vi "Configure Serial.vi"(8 "error in (no error)":errorcluster, 10 "Baud (115200)":u32=115200, 11 "VISA resource name in":refnum<visa-resource-name>) -> (0 "error out":errorcluster, 3 "VISA resource name":refnum<visa-resource-name>)   [LabVIEW 2023, in "CTI-Visa.lvlib"]
uses:
  CTI-Visa.lvlib
  <vilib>/Instr/_visa.llb/VISA Configure Serial Port (Instr).vi
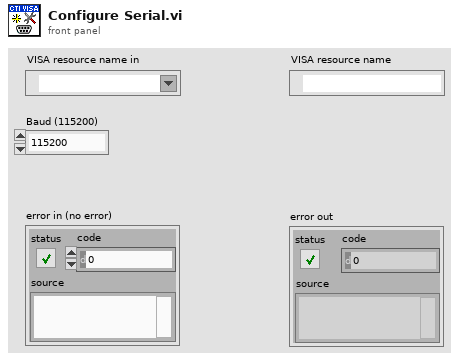
[diagram p1: front panel]
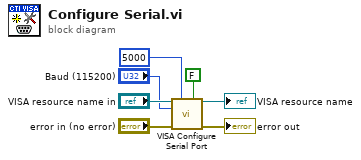
[diagram p0: block diagram]
diagram:
  n1 = call-poly "VISA Configure Serial Port"("VISA resource name"="VISA resource name in", "timeout (10sec)"=u32 5000, "Enable Termination\nChar (T)"=FALSE ("Enable Termination\nChar (T)"), "baud rate (9600)"="Baud (115200)", "error in (no error)"="error in (no error)") -> ("VISA resource name out"=→"VISA resource name":refnum<visa-resource-name>, "error out"=→"error out":errorcluster)  [unwired: 9 in]
